vi "KE22XX_Basic_All_CH_Setting(Modif).vi"(0 "VISA In":refnum<visa-resource-name>, 1 "Channe 1":T1, 2 "Channe 2":T1, 3 "Channe 3":T1, 5 "ID ?":bool, 7 "Remote":bool, 9 "Reset":bool, 11 "error in":errorcluster) -> (15 "error out":errorcluster)   [LabVIEW 2016]
uses:
  Channel Control.ctl
  <userlib>/_TI-LA/Instr Drivers/Power Supply/KE22xx/Driver/Base/Keithley KE22xx Series.lvlib
panel:
  in  "Tab Control":enum32{"Channel 1", "Channel 2", "Channel 3"}(tab)
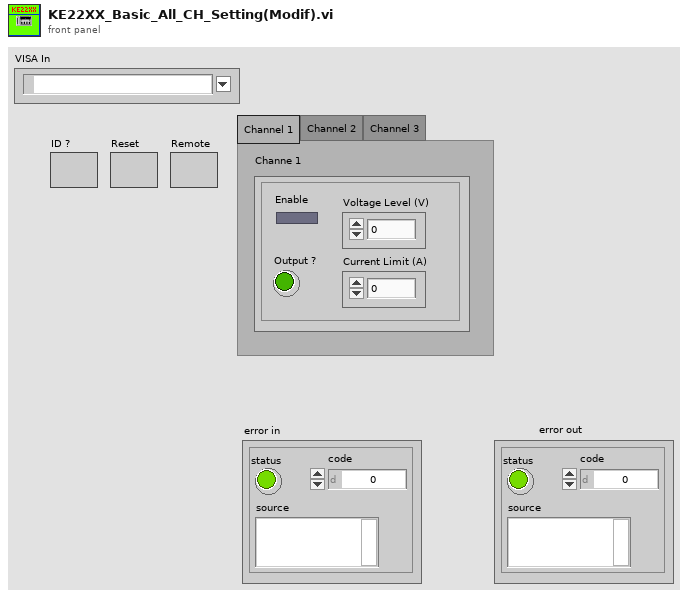
[diagram p1: front panel]
types:
  T1 = typedef "Channel Control.ctl" = cluster{"Output ?":bool, "Enable":bool, "Voltage Level (V)":dbl, "Current Limit (A) ":dbl}
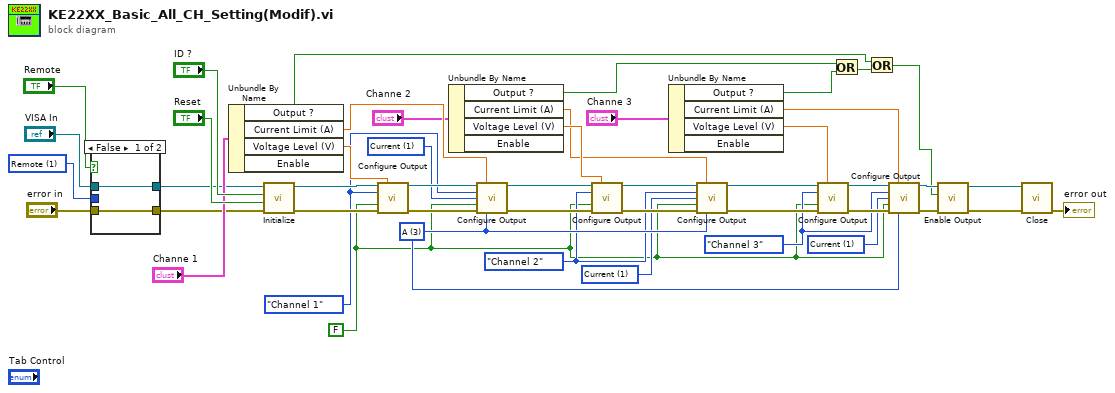
[diagram p0: block diagram]
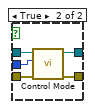
[diagram p2: hidden frame]
diagram:
  w10 = FALSE ("Enable Output (T: Enable)")
  w12 = u16 1 items=["Voltage", "Current"] ("Function(0:Voltage)")
  w11 = enum16{"Channel 1", "Channel 2", "Channel 3"}."Channel 3" ("Channel Select")
  w18 = u16 1 items=["Voltage", "Current"] ("Function(0:Voltage)")
  w17 = enum16{"Channel 1", "Channel 2", "Channel 3"}."Channel 2" ("Channel Select")
  w22 = u16 1 items=["Voltage", "Current"] ("Function(0:Voltage)")
  w21 = enum16{"Channel 1", "Channel 2", "Channel 3"}."Channel 1" ("Channel Select")
  w26 = u16 3 items=["V", "mV", "kV", "A", "mA"] ("Unit(V)")
  w27 = u16 1 items=["Local", "Remote", "Remote Lock"] ("Control Mode (1: Remote)")
  n1 = case shown="False" "Remote" {
    tunnel: [w49 w54] -> w31
    tunnel: "VISA In" -> [w49 w53]
    tunnel: "error in" -> [w48 w52]
    tunnel: [w48 w51] -> w28
    tunnel: w27 -> [_ w50]
    frame False {
    }
    frame True {
      n2 = call <userlib>:"Control Mode.vi"("error in (no error)"=w52, "Control Mode (1: Remote)"=w50, "VISA resource name"=w53) -> ("error out"=w51:errorcluster, "VISA resource name out"=w54:refnum<visa-resource-name>)  [unwired: 7 in]
    }
  }
  n3 = Unbundle By Name("Channe 1") -> ("Output ?"=w2:bool, "Current Limit (A)"=w41:dbl, "Voltage Level (V)"=w42:dbl)  [unwired: 1 out]
  n4 = call <userlib>:"Initialize.vi"("error in (no error)"=w28, "Reset (True)"="Reset", "ID Query (True)"="ID ?", "VISA resource name"=w31) -> ("error out"=w44:errorcluster, "VISA resource name out"=w45:refnum<visa-resource-name>)  [unwired: 6 in]
  n5 = call <userlib>:"Configure Output.vi"("VISA resource name"=w45, "Manual Range(0.00)"=w42, "Channel Select"=w21, "Enable Output (T: Enable)"=w10, "error in (no error)"=w44) -> ("VISA resource name out"=w24:refnum<visa-resource-name>, "error out"=w23:errorcluster)  [unwired: 9 in]
  n6 = Unbundle By Name("Channe 2") -> ("Output ?"=w4:bool, "Current Limit (A)"=w38:dbl, "Voltage Level (V)"=w39:dbl)  [unwired: 1 out]
  n7 = call <userlib>:"Configure Output.vi"("VISA resource name"=w24, "Manual Range(0.00)"=w41, "Channel Select"=w21, "Function(0:Voltage)"=w22, "Enable Output (T: Enable)"=w10, "error in (no error)"=w23, "Unit(V)"=w26) -> ("VISA resource name out"=w37:refnum<visa-resource-name>, "error out"=w36:errorcluster)  [unwired: 7 in]
  n8 = call <userlib>:"Configure Output.vi"("VISA resource name"=w37, "Manual Range(0.00)"=w39, "Channel Select"=w17, "Enable Output (T: Enable)"=w10, "error in (no error)"=w36) -> ("VISA resource name out"=w20:refnum<visa-resource-name>, "error out"=w19:errorcluster)  [unwired: 9 in]
  n9 = Unbundle By Name("Channe 3") -> ("Output ?"=w5:bool, "Current Limit (A)"=w33:dbl, "Voltage Level (V)"=w34:dbl)  [unwired: 1 out]
  n10 = call <userlib>:"Configure Output.vi"("VISA resource name"=w20, "Manual Range(0.00)"=w38, "Channel Select"=w17, "Function(0:Voltage)"=w18, "Enable Output (T: Enable)"=w10, "error in (no error)"=w19, "Unit(V)"=w26) -> ("VISA resource name out"=w15:refnum<visa-resource-name>, "error out"=w16:errorcluster)  [unwired: 7 in]
  n11 = call <userlib>:"Configure Output.vi"("VISA resource name"=w15, "Manual Range(0.00)"=w34, "Channel Select"=w11, "Enable Output (T: Enable)"=w10, "error in (no error)"=w16) -> ("VISA resource name out"=w14:refnum<visa-resource-name>, "error out"=w13:errorcluster)  [unwired: 9 in]
  n12 = Or(x=w4, y=w5) -> (x .or. y?=w3:bool)
  n13 = Or(x=w2, y=w3) -> (x .or. y?=w1:bool)
  n14 = call <userlib>:"Configure Output.vi"("VISA resource name"=w14, "Manual Range(0.00)"=w33, "Channel Select"=w11, "Function(0:Voltage)"=w12, "Enable Output (T: Enable)"=w10, "error in (no error)"=w13, "Unit(V)"=w26) -> ("VISA resource name out"=w9:refnum<visa-resource-name>, "error out"=w8:errorcluster)  [unwired: 7 in]
  n15 = call <userlib>:"Enable Output.vi"("error in (no error)"=w8, "Enable Output (T: Enable)"=w1, "VISA resource name"=w9) -> ("error out"=w7:errorcluster, "VISA resource name out"=w6:refnum<visa-resource-name>)  [unwired: 7 in]
  n16 = call <userlib>:"Close.vi"("error in (no error)"=w7, "VISA resource name"=w6) -> ("error out"=→"error out":errorcluster)  [unwired: 9 in]
